vi "Dictionary Filter by In Word.vi"(10 "Words_Ref in":refnum<vi>[](array[refnum]), 11 "Dictionary in":string[](array[string])) -> (3 "Dictionary out":string[](array[string]))   [LabVIEW 2015]
uses:
  TypeDef/Color.ctl
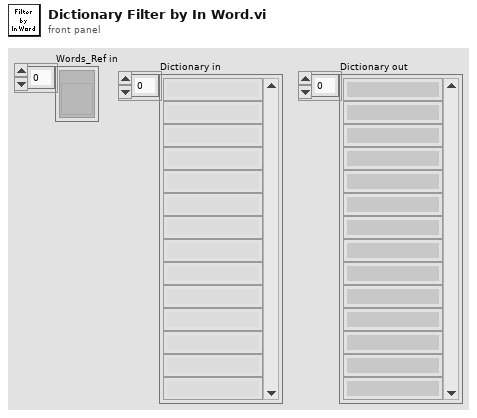
[diagram p1: front panel]
types:
  T1 = typedef "Color.ctl" = u32
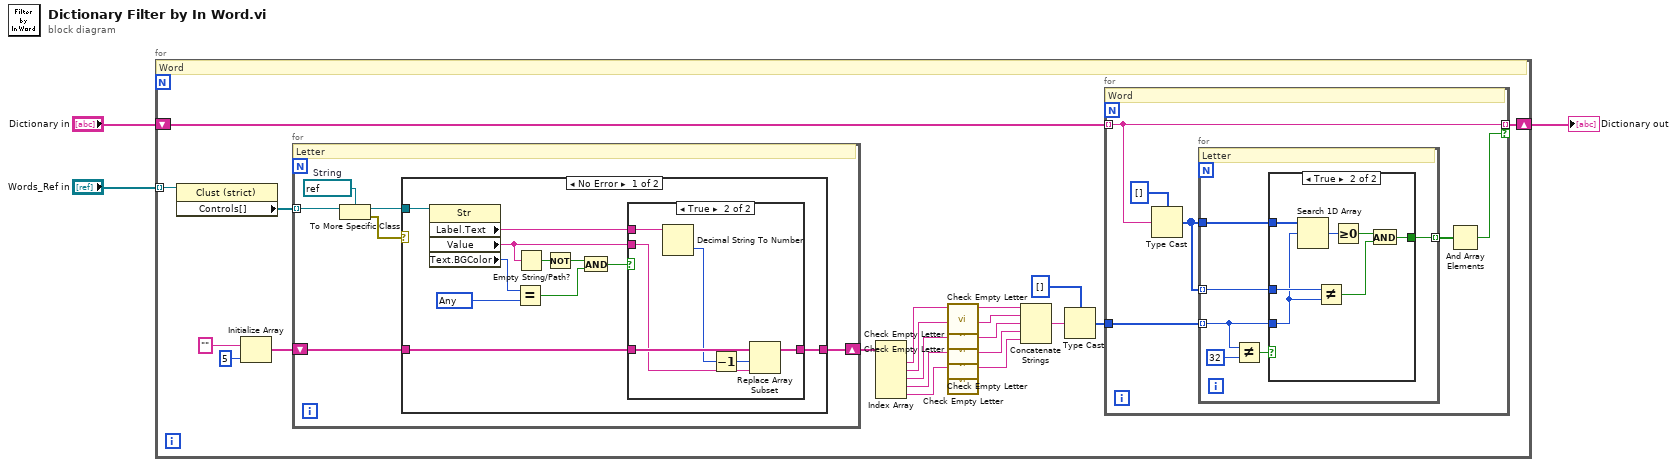
[diagram p0: block diagram]
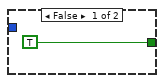
[diagram p4: hidden frame]
diagram:
  n1 = for {
    tunnel: "Words_Ref in" -> [w23] mode=indexing
    shift-right: [w10] -> w1
    shift-left: "Dictionary in" -> [w11]
    # "Word"
    n2 = property class="Clust (strict)"(reference=w23) -> ("Controls[]"=w24:refnum<vi>[])  [unwired: 1 in, 2 out]
    n3 = Initialize Array("", 5 ("dimension size")) -> (w20:string[])
    n4 = for {
      tunnel: w24 -> [w28] mode=indexing
      shift-right: [w29] -> w9
      shift-left: w20 -> [w30]
      w26 = refnum<vi> refnum  # String
      # "Letter"
      n5 = To More Specific Class(target class=w26, reference=w28) -> (specific class reference=w27:refnum<vi>, error out=w25:errorcluster)  [unwired: 1 in]
      n6 = case shown="No Error" w25 {
        tunnel: w30 -> [w40 w49]
        tunnel: [w39 w49] -> w29
        tunnel: w27 -> [w38 _]
        frame No Error {
          w35 = T1 16448250 items=["Free"=9567230, "Letter"=16774186, "Any"=16448250, "Exclude"=12369084] ("Color")
          n7 = property class="Str"(reference=w38) -> ("Label.Text"=w41:string, "Value"=w31:string, "Text.BGColor"=w36:u32)  [unwired: 1 in, 2 out]
          n8 = Equal?(x=w36, y=w35) -> (x = y?=w33:bool)
          n9 = Empty String/Path?(string/path=w31) -> (empty?=w37:bool)
          n10 = Not(x=w37) -> (.not. x?=w34:bool)
          n11 = And(x=w34, y=w33) -> (x .and. y?=w32:bool)
          n12 = case shown="True" w32 {
            tunnel: w41 -> [_ w48]
            tunnel: w40 -> [w42 w47]
            tunnel: [w42 w46] -> w39
            tunnel: w31 -> [_ w43]
            frame False {
            }
            frame True {
              n13 = Decimal String To Number(string=w48) -> (number=w45:i32)  [unwired: 2 in, 1 out]
              n14 = Decrement(x=w45) -> (x-1=w44:i32)
              n15 = Replace Array Subset(array=w47, new element=w43, index=w44) -> (w46:string[])
            }
          }
        }
        frame Error {
        }
      }
    }
    n16 = Index Array(array=w9) -> (element #1=w8:string, element #2=w7:string, element #3=w6:string, element #4=w5:string, element #5=w4:string)  [unwired: 5 in]
    n17 = call "Check Empty Letter.vi"("Letter in"=w8) -> ("Letter Out"=w14:string)  [unwired: 10 in]
    n18 = call "Check Empty Letter.vi"("Letter in"=w7) -> ("Letter Out"=w15:string)  [unwired: 10 in]
    n19 = call "Check Empty Letter.vi"("Letter in"=w6) -> ("Letter Out"=w16:string)  [unwired: 10 in]
    n20 = call "Check Empty Letter.vi"("Letter in"=w5) -> ("Letter Out"=w17:string)  [unwired: 10 in]
    n21 = call "Check Empty Letter.vi"("Letter in"=w4) -> ("Letter Out"=w18:string)  [unwired: 10 in]
    n22 = Concatenate Strings(w14, w15, w16, w17, w18) -> (w12:string)
    n23 = Type Cast(type=u8[] [], x=w12) -> (*(type *) &x=w19:u8[])
    n24 = for {
      tunnel: w19 -> [w55]
      tunnel: w11 -> [w53] mode=indexing
      tunnel: [w53] -> w10 mode=indexing if=w51
      # "Word"
      n25 = Type Cast(type=u8[] [], x=w53) -> (*(type *) &x=w50:u8[])
      n26 = for {
        tunnel: w55 -> [w58] mode=indexing
        tunnel: w50 -> [w61]
        tunnel: [w60] -> w52 mode=indexing
        tunnel: w50 -> [w56] mode=indexing
        # "Letter"
        n27 = Not Equal?(x=w58, y=u8 32) -> (x != y?=w59:bool)
        n28 = case shown="True" w59 {
          tunnel: w61 -> [_ w69]
          tunnel: w58 -> [_ w65]
          tunnel: [TRUE w64] -> w60
          tunnel: w56 -> [_ w66]
          frame False {
          }
          frame True {
            n29 = Search 1D Array(1D array=w69, element=w65) -> (index of element=w68:i32)  [unwired: 1 in]
            n30 = Not Equal?(x=w66, y=w65) -> (x != y?=w63:bool)
            n31 = Greater Or Equal To 0?(x=w68) -> (x >= 0?=w67:bool)
            n32 = And(x=w67, y=w63) -> (x .and. y?=w64:bool)
          }
        }
      }
      n33 = And Array Elements(Boolean array=w52) -> (logical AND=w51:bool)
    }
  }
  "Dictionary out" <- w1
